vi "fpga-main.vi"() -> ()   [LabVIEW 2020]
doc: "This VI measures the high and low periods of a pulse width modulated signal."
uses:
  <vilib>/rvi/Emulation/niFpgaGetClockAttributes.vi
  <vilib>/rvi/Emulation/niFpgaSctlEmulationGetInTimedLoop.vi
  <vilib>/rvi/Emulation/niFpgaEmulationReportErrorSimple.vi
  <vilib>/rvi/interface/RandomDataEmulation/nirviRandomDataMultiElementFPGAFIFO.vi
  <instcachedir>/0/nirviRandomDataMultiElementFPGAFIFO_3E9965BA1FAD4E7B8DABA31768A09B1F.lvgen/nirviRandomDataMultiElementFPGAFIFO_3E9965BA1FAD4E7B8DABA31768A09B1F_001.vi
  <vilib>/rvi/interface/RandomDataEmulation/niFpgaRandomDataHandleErrors.vi
  <vilib>/rvi/eio/common/nirviEmuTemplateMethod_errors.vi
  <vilib>/rvi/Emulation/niFpgaCriticalErrorInLSC.vi
  <vilib>/rvi/DataTransferAndStorage/Container/XNode/niFpgaContainer.xnode
  <vilib>/rvi/interface/RandomDataEmulation/nirviRandomDataFpgaMultiElementTemplate.vi
  <vilib>/eio/EIONode/EIONode.xnode
  <vilib>/LabVIEW Targets/FPGA/RIO/nicrio_985x_controls.llb/CAN_IO_Frame Array U32.ctl
panel:
  out "CAN1_Tx":u32[](array[numeric]) format="%.0x"
  out "CAN1_Rx":u32[](array[numeric]) format="%.0x"
  out "CAN0_Tx":u32[](array[numeric]) format="%.0x"
  out "CAN0_Rx":u32[](array[numeric]) format="%.0x"
  # "CAN Debug Panel"
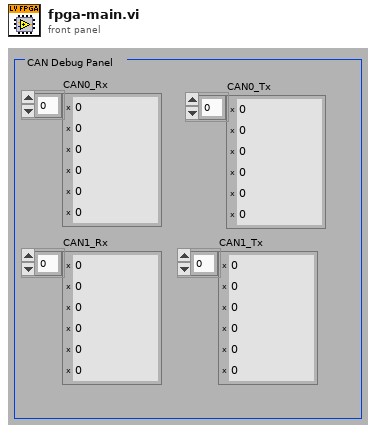
[diagram p1: front panel]
types:
  T1 = typedef "CAN_IO_Frame Array U32.ctl" = u32[]
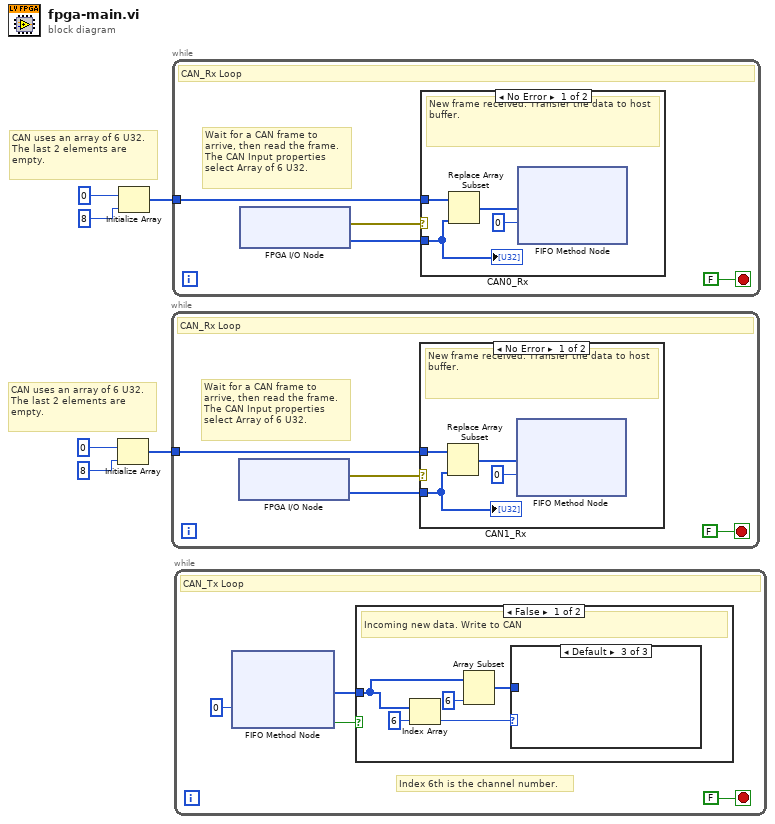
[diagram p0: block diagram]
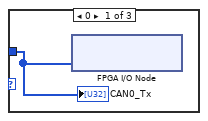
[diagram p3: hidden frame]
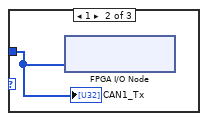
[diagram p4: hidden frame]
diagram:
  # "CAN uses an array of 6 U32. The last 2 elements are empty."
  # "CAN uses an array of 6 U32. The last 2 elements are empty."
  n1 = Initialize Array(u32 0 ("U32"), 8 ("Number of Elements to Read")) -> (w3:u32[])
  n2 = Initialize Array(u32 0 ("U32"), 8 ("Number of Elements to Read")) -> (w4:u32[])
  n3 = while {
    tunnel: w3 -> [w7]
    stop <- FALSE stop-if-true
    # "Wait for a CAN frame to\narrive, then read the frame. \nThe CAN Input properties \nselect Array of 6 U32."
    # "CAN_Rx Loop"
    n4 = xnode "FPGA I/O Node"() -> ("error out"=w9:errorcluster, "Mod8/CAN1"=w8:T1)  [unwired: 2 in, 1 out]
    n5 = case shown="No Error" w9 {
      tunnel: w8 -> [w12 _]
      tunnel: w7 -> [w13 _]
      frame No Error {
        # "New frame received. Transfer the data to host buffer."
        n6 = Replace Array Subset(array=w13, new element=w12) -> (w11:u32[])  [unwired: 1 in]
        n7 = xnode ("FIFO Method Node")("Element"=w11, "Timeout"=0) -> ()  [unwired: 1 in, 2 out]
        "CAN1_Rx" <- w12
      }
      frame Error {
        # "No new frame. Do nothing."
      }
    }
  }
  n8 = while {
    tunnel: w4 -> [w15]
    stop <- FALSE stop-if-true
    # "Wait for a CAN frame to\narrive, then read the frame. \nThe CAN Input properties \nselect Array of 6 U32."
    # "CAN_Rx Loop"
    n9 = xnode "FPGA I/O Node"() -> ("error out"=w17:errorcluster, "Mod8/CAN0"=w16:T1)  [unwired: 2 in, 1 out]
    n10 = case shown="No Error" w17 {
      tunnel: w16 -> [w20 _]
      tunnel: w15 -> [w21 _]
      frame No Error {
        # "New frame received. Transfer the data to host buffer."
        n11 = Replace Array Subset(array=w21, new element=w20) -> (w19:u32[])  [unwired: 1 in]
        n12 = xnode ("FIFO Method Node")("Element"=w19, "Timeout"=0) -> ()  [unwired: 1 in, 2 out]
        "CAN0_Rx" <- w20
      }
      frame Error {
        # "No new frame. Do nothing."
      }
    }
  }
  n13 = while {
    stop <- FALSE stop-if-true
    # "Index 6th is the channel number."
    # "CAN_Tx Loop"
    n14 = xnode ("FIFO Method Node")("Timeout"=0) -> ("Element"=w23:u32[], "Timed Out?"=w24:bool)  [unwired: 1 in, 1 out]
    n15 = case shown="False" w24 {
      tunnel: w23 -> [w31 _]
      frame False {
        # "Incoming new data. Write to CAN"
        n16 = Index Array(array=w31, index=6) -> (element=w29:u32)
        n17 = Array Subset(array=w31, length=6) -> (w27:u32[])  [unwired: 1 in]
        n18 = case shown="Default" w29 {
          tunnel: w27 -> [w32 w33 _]
          frame 0 {
            n19 = xnode "FPGA I/O Node"("Mod8/CAN0"=w32) -> ()  [unwired: 1 in, 1 out]
            "CAN0_Tx" <- w32
          }
          frame 1 {
            n20 = xnode "FPGA I/O Node"("Mod8/CAN1"=w33) -> ()  [unwired: 1 in, 1 out]
            "CAN1_Tx" <- w33
          }
          frame Default {
          }
        }
      }
      frame True {
        # "Timeout, no new data. Do nothing."
      }
    }
  }
